vi "niRFUtil WFM Compensate IQ Quadrature Error.vi"(0 "Input":T1 {"y" format="%.2f"; "dx" format="%^.2e"; "x0" format="%^.2e"}, 7 "Phase Imbalance (rad)":sgl, 11 "Compensate?":bool) -> (4 "Waveform Out":T1 {"y" format="%.2f"; "dx" format="%^.2e"; "x0" format="%^.2e"})   [LabVIEW 2015, in "niRFUtil.lvlib"]
uses:
  niRFUtil.lvlib
  Includes/niRFUtil INC Complex Waveform.ctl
  Includes/niRFUtil INC Complex Array.ctl
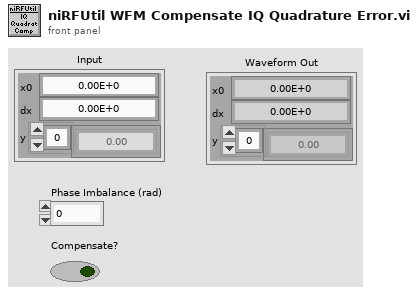
[diagram p1: front panel]
types:
  T1 = typedef "niRFUtil.lvlib/niRFUtil INC Complex Waveform.ctl" = cluster{"x0":dbl, "dx":dbl, "y":T2}
  T2 = typedef "niRFUtil.lvlib/niRFUtil INC Complex Array.ctl" = csg[]
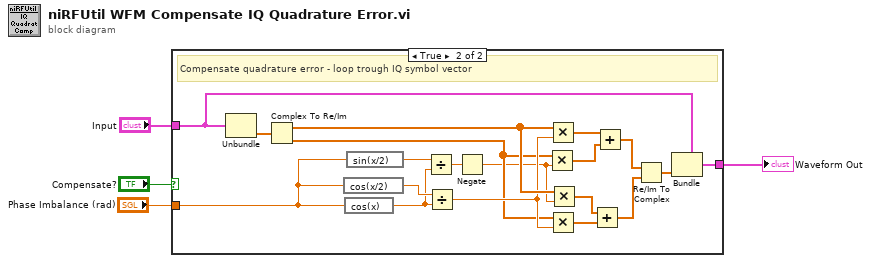
[diagram p0: block diagram]
diagram:
  n1 = case shown="True" "Compensate?" {
    tunnel: "Input" -> [w5 w22]
    tunnel: [w5 w23] -> w4
    tunnel: "Phase Imbalance (rad)" -> [_ w13]
    frame False {
    }
    frame True {
      # "Compensate quadrature error - loop trough IQ symbol vector"
      n2 = Unbundle(w22) -> ("y"=w24:T2)  [unwired: 2 out]
      n3 = Complex To Re/Im(x + iy=w24) -> (x=w9:sgl[], y=w7:sgl[])
      n4 = expression code="cos(x/2)"(w13) -> (w20:sgl)
      n5 = expression code="cos(x)"(w13) -> (w19:sgl)
      n6 = expression code="sin(x/2)"(w13) -> (w21:sgl)
      n7 = Divide(x=w21, y=w19) -> (x/y=w18:sgl)
      n8 = Divide(x=w20, y=w19) -> (x/y=w8:sgl)
      n9 = Negate(x=w18) -> (-x=w6:sgl)
      n10 = Multiply(x=w7, y=w6) -> (x*y=w12:sgl[])
      n11 = Multiply(x=w9, y=w8) -> (x*y=w11:sgl[])
      n12 = Multiply(x=w7, y=w8) -> (x*y=w16:sgl[])
      n13 = Multiply(x=w9, y=w6) -> (x*y=w17:sgl[])
      n14 = Add(x=w17, y=w16) -> (x+y=w14:sgl[])
      n15 = Add(x=w11, y=w12) -> (x+y=w15:sgl[])
      n16 = Re/Im To Complex(1:w14, 2:w15) -> (0:w10:csg[])
      n17 = Bundle(cluster=w22, "y"=w10) -> (w23:T1)  [unwired: 2 in]
    }
  }
  "Waveform Out" <- w4
